vi "WSVCAP SHL FPGA LL Procedure I2C - Send ACK.vi"(0 "Procedure Step":T1, 1 "Wait Ticks Remaining":u32, 5 "I2C Wait Ticks":u32, 7 "ACK Bit to Write":bool, 11 "error in (no error)":errorcluster, 13 "Socket Mask":u64 format="%012x", 14 "UUT (0/1)":u8) -> (3 "Wait Ticks Remaining Out":u32, 4 "Procedure Step Out":T1, 8 "Finished":bool, 15 "error out":errorcluster)   [LabVIEW 2012]
uses:
  Type Defs/WSVCAP SHL Procedure Step Enum.ctl
  Type Defs/WSVCAP SHL I2C Write Line Enum.ctl
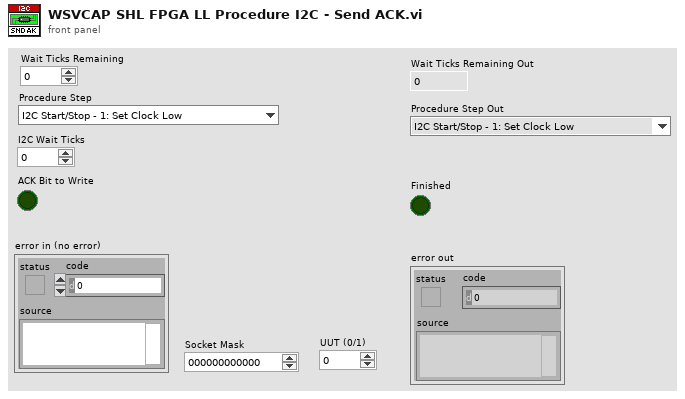
[diagram p1: front panel]
types:
  T1 = typedef "WSVCAP SHL Procedure Step Enum.ctl" = enum16{"I2C Start/Stop - 1: Set Clock Low", "I2C Start/Stop - 2: Wait", "I2C Start/Stop - 3: Set Data I", "I2C Start/Stop - 4: Wait", "I2C Start/Stop - 5: Set Clock High", "I2C Start/Stop - 6: Wait", "I2C Start/Stop - 7: Set Data II", "I2C Start/Stop - 8: Wait", "I2C Start/Stop - 9: Set Clock Low", "I2C Start/Stop - 10: Wait", "I2C Read ACK - 1: Set Clock High", "I2C Read ACK - 2: Wait", "I2C Read ACK - 3: Read ACK Bit", "I2C Read ACK - 4: Wait", "I2C Read ACK - 5: Set Clock Low", "I2C Read ACK - 6: Wait", "I2C Write ACK - 1: Write ACK Bit", "I2C Write ACK - 2: Wait", "I2C Write ACK - 3: Set Clock High", "I2C Write ACK - 4: Wait", "I2C Write ACK - 5: Set Clock Low", "I2C Write ACK - 6: Wait", "I2C Write ACK - 7: Set Data Low", "I2C Send Add - 1: Reset Bits Remaining", "I2C Send Add - 2: Set Data Bit", "I2C Send Add - 3: Wait", "I2C Send Add - 4: Set Clock High", "I2C Send Add - 5: Wait", "I2C Send Add - 6: Set Clock Low", "I2C Send Add - 7: Wait", "I2C Send Add - 8: Check Bits Remaining", "I2C Send Data - 1: Reset Bits Remaining", "I2C Send Data - 2: Load Write Bit from FIFO", "I2C Send Data - 3: Set Data Bit", "I2C Send Data - 4: Wait", "I2C Send Data - 5: Set Clock High", "I2C Send Data - 6: Wait", "I2C Send Data - 7: Set Clock Low", "I2C Send Data - 8: Wait", "I2C Send Data - 9: Check Bits Remaining", "I2C Receive Data - 1: Reset Bits Remaining", "I2C Receive Data - 2: Wait", "I2C Receive Data - 3: Set Clock High", "I2C Receive Data - 4: Wait", "I2C Receive Data - 5: Read Data Bit", "I2C Receive Data - 6: Wait", "I2C Receive Data - 7: Set Clock Low", "I2C Receive Data - 8: Wait", "I2C Receive Data - 9: Check Bits Remaining", "RFFE Send SSC - 1:Set Low", "RFFE Send SSC - 2:Wait", "RFFE Send SSC - 3:Set SDA High", "RFFE Send SSC - 4:Wait", "RFFE Send SSC - 5:Set SDA Low", "RFFE Send SSC - 6:Wait", "RFFE Send Data - 1:Set SCL High", "RFFE Send Data - 2:Wait", "RFFE Send Data - 3:Set SCL Low", "RFFE Send Data - 4:Wait", "RFFE Send Data - 5:Set SCL High (P)", "RFFE Send Data - 6:Wait", "RFFE Send Data - 7:Set SCL Low (P)", "RFFE Send Data - 8:Wait", "RFFE Send Data - 9:Set SCL High (BP)", "RFFE Send Data - 10:Wait", "RFFE Send Data - 11:Set SCL Low (BP)", "RFFE Send Data - 12:Wait", "RFFE Receive Data - 1:Set SCL High", "RFFE Receive Data - 2:Wait", "RFFE Receive Data - 3:Set SCL Low", "RFFE Receive Data - 4:Wait", "RFFE Receive Data - 5:Set SCL High (BP)", "RFFE Receive Data - 6:Wait", "RFFE Receive Data - 7:Set SCL Low (BP)", "RFFE Receive Data - 8:Wait", "RFFE Wait CMD Delay - 1:Wait", "RFFE Clear Lines - 1:Clear"}
  T2 = typedef "WSVCAP SHL I2C Write Line Enum.ctl" = enum16{"I2C SCL", "I2C SDA"}
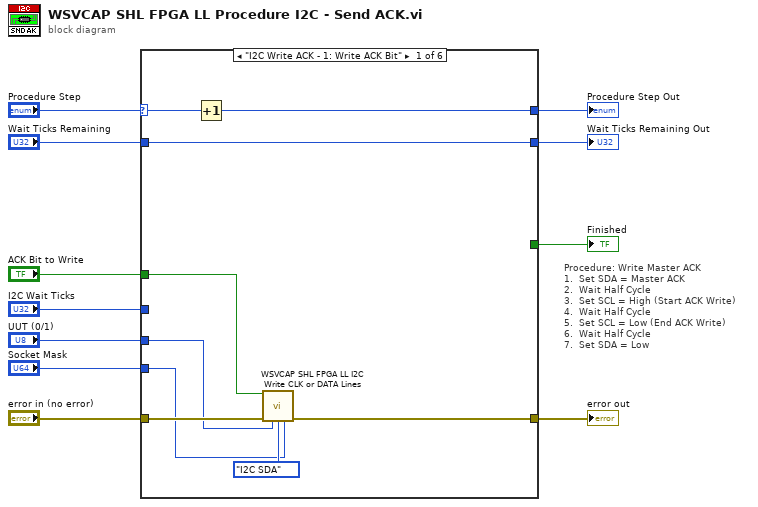
[diagram p0: block diagram]
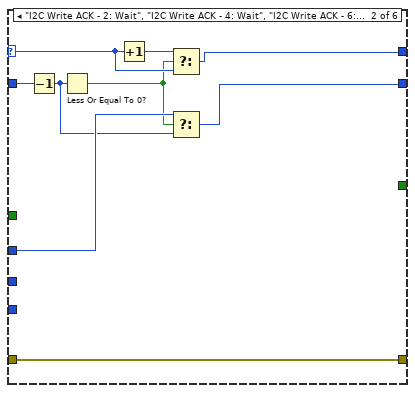
[diagram p2: hidden frame]
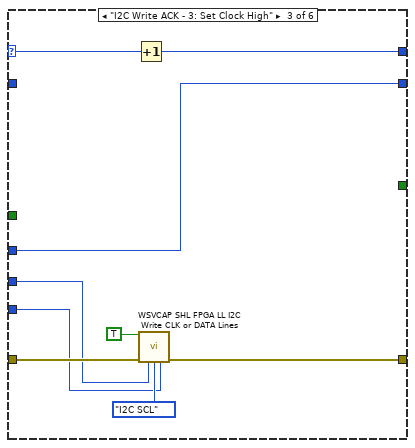
[diagram p3: hidden frame]
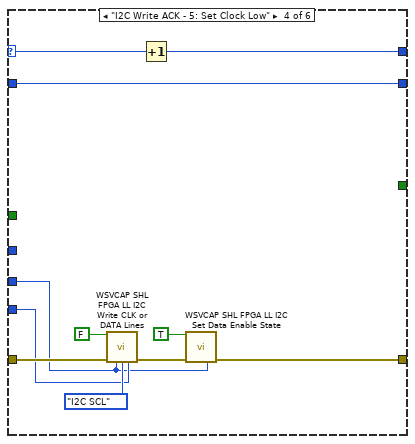
[diagram p4: hidden frame]
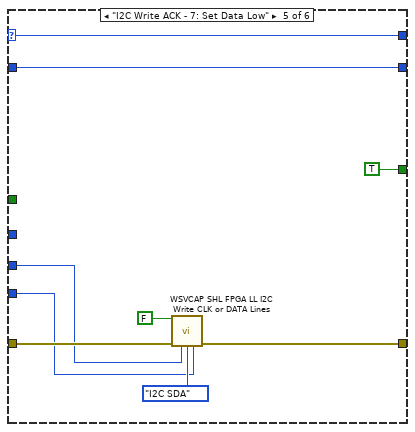
[diagram p5: hidden frame]
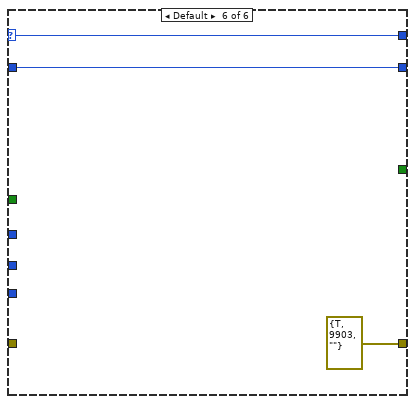
[diagram p6: hidden frame]
diagram:
  # "Procedure: Write Master ACK\n1.  Set SDA = Master ACK\n2.  Wait Half Cycle\n3.  Set SCL = High (Start ACK Write)\n4.  Wait Half Cycle\n5.  Set SCL = Low (End ACK Write)\n6.  Wait Half Cycle\n7.  Set SDA = Low"
  n1 = case shown="\"I2C Write ACK - 1: Write ACK Bit\"" "Procedure Step" {
    selector: "Procedure Step" -> [w18 w24 w35 w43 w52 w60]
    tunnel: [w19 w27 w34 w45 w55 errorcluster {"status"=TRUE, "code"=9903, "source"=""} ("error out")] -> w10
    tunnel: "error in (no error)" -> [w20 w27 w37 w48 w56 _]
    tunnel: "Wait Ticks Remaining" -> [w13 w29 _ w40 w51 w59]
    tunnel: "I2C Wait Ticks" -> [_ w26 w31 _ _ _]
    tunnel: [_ _ _ _ TRUE _] -> w9
    tunnel: "ACK Bit to Write" -> [w17 _ _ _ _ _]
    tunnel: "Socket Mask" -> [w15 _ w33 w42 w53 _]
    tunnel: [w14 w22 w32 w41 w52 w60] -> w3
    tunnel: [w13 w21 w31 w40 w51 w59] -> w2
    tunnel: "UUT (0/1)" -> [w12 _ w30 w39 w50 _]
    frame "I2C Write ACK - 1: Write ACK Bit" {
      n2 = Increment(x=w18) -> (x+1=w14:T1)
      n3 = call "WSVCAP SHL FPGA LL I2C Write CLK or DATA Lines.vi"("Bit In"=w17, "error in (no error)"=w20, "UUT Set (0/1)"=w12, "Line"=WSVCAP_SHL_I2C_Write_Line_Enum."I2C SDA", "Socket Mask"=w15) -> ("error out"=w19:errorcluster)  [unwired: 10 in]
    }
    frame "I2C Write ACK - 2: Wait", "I2C Write ACK - 4: Wait", "I2C Write ACK - 6: Wait" {
      n4 = Decrement(x=w29) -> (x-1=w25:u32)
      n5 = Less Or Equal To 0?(x=w25) -> (x <= 0?=w23:bool)
      n6 = Increment(x=w24) -> (x+1=w28:T1)
      n7 = Select(t=w28, s=w23, f=w24) -> (s? t:f=w22:T1)
      n8 = Select(t=w26, s=w23, f=w25) -> (s? t:f=w21:u32)
    }
    frame "I2C Write ACK - 3: Set Clock High" {
      n9 = Increment(x=w35) -> (x+1=w32:T1)
      n10 = call "WSVCAP SHL FPGA LL I2C Write CLK or DATA Lines.vi"("Bit In"=TRUE, "error in (no error)"=w37, "UUT Set (0/1)"=w30, "Line"=WSVCAP_SHL_I2C_Write_Line_Enum."I2C SCL", "Socket Mask"=w33) -> ("error out"=w34:errorcluster)  [unwired: 10 in]
    }
    frame "I2C Write ACK - 5: Set Clock Low" {
      n11 = call "WSVCAP SHL FPGA LL I2C Write CLK or DATA Lines.vi"("Bit In"=FALSE, "error in (no error)"=w48, "UUT Set (0/1)"=w39, "Line"=WSVCAP_SHL_I2C_Write_Line_Enum."I2C SCL", "Socket Mask"=w42) -> ("error out"=w46:errorcluster)  [unwired: 10 in]
      n12 = Increment(x=w43) -> (x+1=w41:T1)
      n13 = call "WSVCAP SHL FPGA LL I2C Set Data Enable State.vi"("State"=TRUE, "error in (no error)"=w46, "UUT Set (0/1)"=w39) -> ("error out"=w45:errorcluster)  [unwired: 12 in]
    }
    frame "I2C Write ACK - 7: Set Data Low" {
      n14 = call "WSVCAP SHL FPGA LL I2C Write CLK or DATA Lines.vi"("Bit In"=FALSE, "error in (no error)"=w56, "UUT Set (0/1)"=w50, "Line"=WSVCAP_SHL_I2C_Write_Line_Enum."I2C SDA", "Socket Mask"=w53) -> ("error out"=w55:errorcluster)  [unwired: 10 in]
    }
    frame Default {
    }
  }
  "error out" <- w10
  "Finished" <- w9
  "Procedure Step Out" <- w3
  "Wait Ticks Remaining Out" <- w2
